vi "RCServo example.vi"() -> ()   [LabVIEW 2012, in "Phidget RC Servo.lvlib"]
uses:
  <instrlib>/Phidgets/Phidget RC Servo/Phidget RC Servo.lvlib
  <instrlib>/Phidgets/Phidget RC Servo/Public/RCServoStart.vi
  <instrlib>/Phidgets/Phidget RC Servo/Public/RCServoClose.vi
  <instrlib>/Phidgets/Phidget Common/Phidget Common.lvlib
panel:
  in  "RCServo Initialization Data":T1={"Velocity Limit"=180.0, "Acceleration"=360.0, "Min PW"=550.0, "Max PW"=2350.0, "Max Position"=180.0, "Min Position"=0.0, "Speed Ramping State"=TRUE}
  out "Position":dbl
  in  "Device Info":T2={"Serial Number"=-1, "Channel"=0, "Port"=0}
  out "Moving":bool
  in  "Engaged":bool=TRUE
  in  "STOP":bool
  in  "Target Position":dbl(slide) scale=0.0..180.0 scale format="%#_2f"
  out "Attached?":bool
  out "Serial Number Return":i32
  out "error out":errorcluster
  # "Be sure to use this stop button to stop the program.\nIf you use the \"Abort Execution\" button, you will\nneed to use PhidgetResetLibrary.vi or restart Labview \nin order for any Phidgets to work."
  # "Enabled\n\nDisabled"
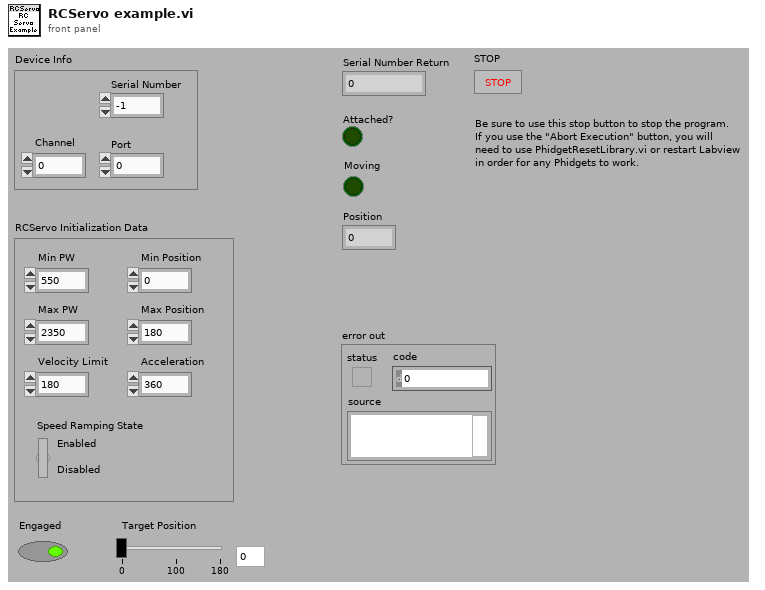
[diagram p1: front panel]
types:
  T1 = cluster{"Velocity Limit":dbl, "Acceleration":dbl, "Min PW":dbl, "Max PW":dbl, "Max Position":dbl, "Min Position":dbl, "Speed Ramping State":bool}
  T2 = cluster{"Serial Number":i32, "Channel":i32, "Port":i32}
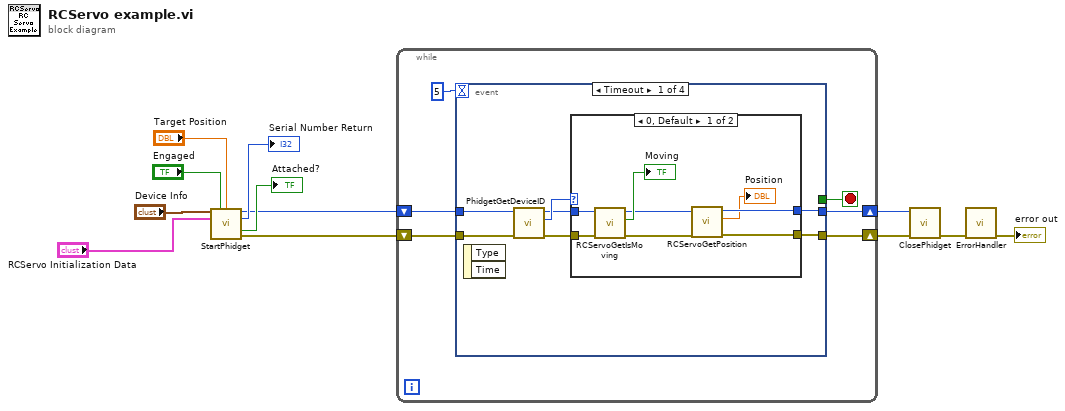
[diagram p0: block diagram]
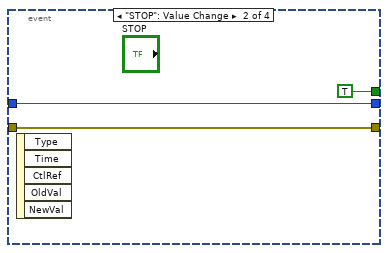
[diagram p3: hidden frame]
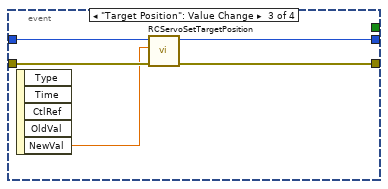
[diagram p4: hidden frame]
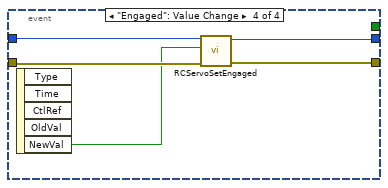
[diagram p5: hidden frame]
diagram:
  n1 = call-poly <instrlib>:"StartPhidget.vi"("Device Info"="Device Info", "Engaged"="Engaged", "Target Position"="Target Position", "RCServo Initialization Data"="RCServo Initialization Data") -> ("Phidget ID"=w1:u64, "Serial Number Return"=→"Serial Number Return":i32, "Attached?"=→"Attached?":bool, "error out"=w2:errorcluster)  [unwired: 8 in]
  n2 = while {
    shift-right: [w15] -> w8
    shift-left: w1 -> [w18]
    shift-right: [w16] -> w9
    shift-left: w2 -> [w17]
    stop <- w13 stop-if-true
    n3 = event shown="[0] Timeout" {
      selector: _ -> [_ _ _ _]
      dyn-events: _ -> [_ _ _ _]
      timeout: 5 -> [_ _ _ _]
      tunnel: w18 -> [w23 w37 w43 w48]
      tunnel: w17 -> [w22 w36 w42 w45]
      tunnel: [w24 w36 w41 w46] -> w16
      tunnel: [w25 w37 w40 w47] -> w15
      tunnel: [_ TRUE ("Stop") _ _] -> w13
      event Timeout {
        n4 = event-data() -> ()  [unwired: 1 in, 2 out]
        n5 = call <instrlib>:"PhidgetGetDeviceID.vi"("error in (no error)"=w22, "Device In"=w23) -> ("error out"=w19:errorcluster, "Devie IDs"=w21:u32, "Device Out"=w20:u64)  [unwired: 6 in]
        n6 = case shown="0, Default" w21 {
          tunnel: [w30 w35] -> w25
          tunnel: [w28 w34] -> w24
          tunnel: w20 -> [w27 w35]
          tunnel: w19 -> [w26 w34]
          frame 0, Default {
            n7 = call <instrlib>:"RCServoGetIsMoving.vi"("error in (no error)"=w26, "Device In"=w27) -> ("error out"=w32:errorcluster, "Is Moving"=→"Moving":bool, "Device Out"=w31:u64)  [unwired: 6 in]
            n8 = call <instrlib>:"RCServoGetPosition.vi"("error in (no error)"=w32, "Device In"=w31) -> ("error out"=w28:errorcluster, "Position"=→"Position":dbl, "Device Out"=w30:u64)  [unwired: 6 in]
          }
          frame 2, 3 {
            # "1000, 1001"
          }
        }
      }
      event "STOP": Value Change {
        n9 = event-data() -> ()  [unwired: 1 in, 5 out]
      }
      event "Target Position": Value Change {
        n10 = event-data() -> ("NewVal"=w39:dbl)  [unwired: 1 in, 4 out]
        n11 = call <instrlib>:"RCServoSetTargetPosition.vi"("error in (no error)"=w42, "Target Position"=w39, "Device In"=w43) -> ("error out"=w41:errorcluster, "Device Out"=w40:u64)  [unwired: 6 in]
      }
      event "Engaged": Value Change {
        n12 = event-data() -> ("NewVal"=w44:bool)  [unwired: 1 in, 4 out]
        n13 = call <instrlib>:"RCServoSetEngaged.vi"("error in (no error)"=w45, "Engaged"=w44, "Device In"=w48) -> ("error out"=w46:errorcluster, "Device Out"=w47:u64)  [unwired: 6 in]
      }
    }
  }
  n14 = call-poly <instrlib>:"ClosePhidget.vi"("error in"=w9, "Device In"=w8) -> ("error out"=w12:errorcluster)  [unwired: 9 in]
  n15 = call <instrlib>:"ErrorHandler.vi"("error in"=w12) -> ("error out"=→"error out":errorcluster)  [unwired: 9 in, 1 out]
